vi "control servos.vi"() -> ()   [LabVIEW 2018]
panel:
  in  "Set Servo Position (0 - 180 degrees) 2":u8(slide)=90 scale=0.0..255.0
  in  "Set Servo Position (0 - 180 degrees)":u8(slide)=90 scale=0.0..255.0
  in  "stop":bool
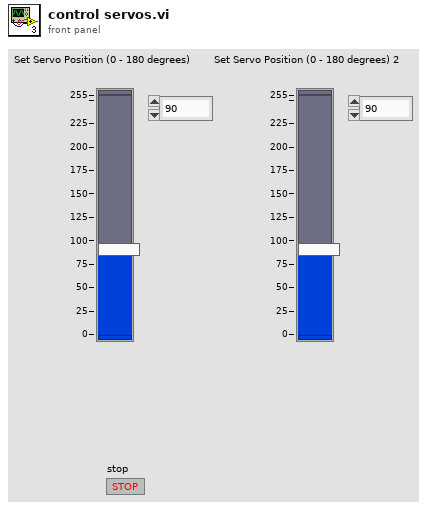
[diagram p1: front panel]
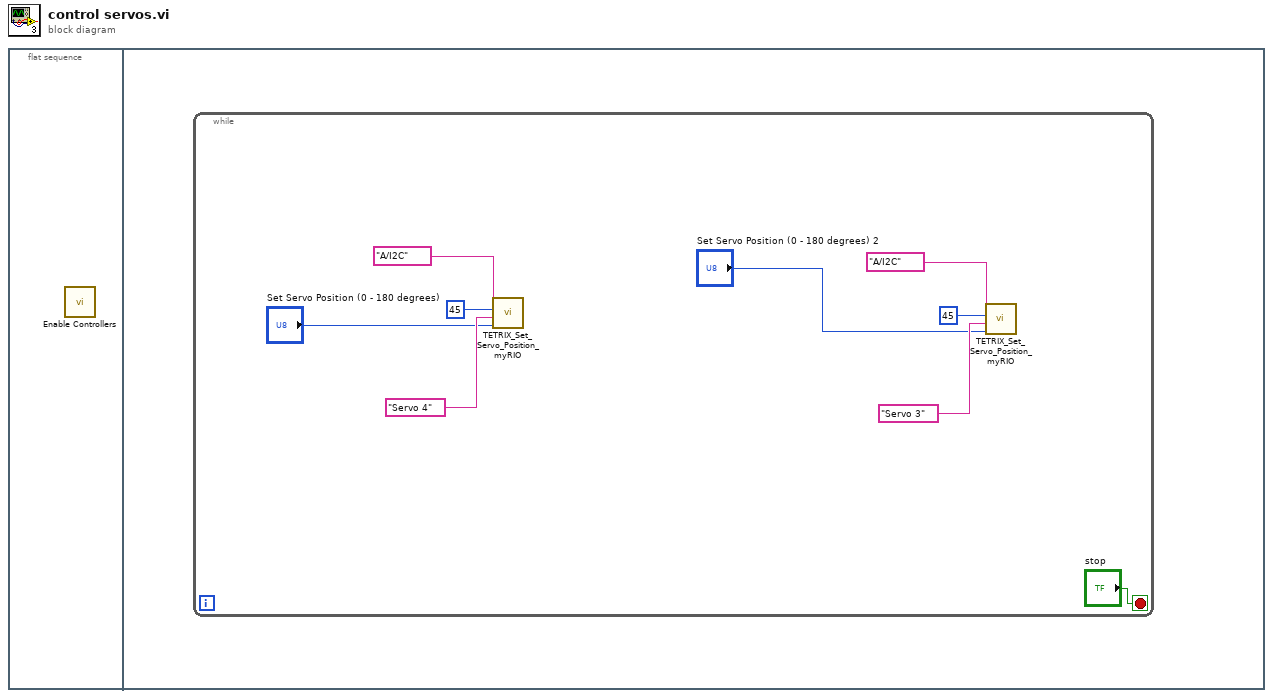
[diagram p0: block diagram]
diagram:
  n1 = flat-sequence {
    frame #0 {
      n2 = call "Enable Controllers.vi"() -> ()  [unwired: 12 in]
    }
    frame #1 {
      n3 = while {
        stop <- "stop" stop-if-true
        n4 = call <vilib>:"TETRIX_Set_Servo_Position_myRIO.vi"("myRIO MXP Port A/B"=tag "A/I2C", "Set Servo Position (0 - 180 degrees)"="Set Servo Position (0 - 180 degrees)", "Select Channel"="Servo 4", "Controller ID#  (I2C Address)"=u8 45) -> ()  [unwired: 3 in, 1 out]
        n5 = call <vilib>:"TETRIX_Set_Servo_Position_myRIO.vi"("myRIO MXP Port A/B"=tag "A/I2C", "Set Servo Position (0 - 180 degrees)"="Set Servo Position (0 - 180 degrees) 2", "Select Channel"="Servo 3", "Controller ID#  (I2C Address)"=u8 45) -> ()  [unwired: 3 in, 1 out]
      }
    }
  }
